vi "niFpga wdp fft tf 4096 U32 inv.vi"(4 "index":fxp<+,11,11>, 10 "enable":bool) -> (2 "imag":fxp<+/-,16,2>, 3 "real":fxp<+/-,16,2>)   [LabVIEW 2017]
uses:
  <vilib>/rvi/Emulation/niFpgaSctlEmulationGetInTimedLoop.vi
  <vilib>/Utility/error.llb/Clear Errors.vi
  <vilib>/rvi/DataTransferAndStorage/Container/Common/niFpgaContainerGetUniqueNameForEmu.vi
  <vilib>/rvi/DataTransferAndStorage/Container/Common/niFpgaContainerSetEmuInfo.vi
  <vilib>/rvi/eio/common/nirviEmuReportErrorAndStop.vi
  <vilib>/rvi/DataTransferAndStorage/Container/Common/niFpgaContainerExecOnDevCompGetState.vi
  <vilib>/rvi/Emulation/niFpgaEmulationIsFPGAContextNoSignature.vi
  <vilib>/rvi/Emulation/niFpgaProcessEmulError.vi
  <vilib>/rvi/errors/nirviReportUnexpectedCaseInternalError (U32).vi
  <vilib>/rvi/Memory/Memory_Emulation/niFpgaMemoryEmulationCacheClearOnFirstRun.vi
  <vilib>/rvi/Memory/Memory_Emulation/nirvimemoryEmulationManagerCache_MakeExclusive.vi
  <vilib>/rvi/Memory/Memory_Emulation/niFpgaMemoryEmulationValidateCache.vi
  <vilib>/rvi/Memory/Memory_Emulation/nirvimemoryEmulationManagerCache_InsertValue.vi
  <vilib>/rvi/Memory/Memory_Emulation/nirvimemoryEmulationManagerCache_ReleaseExclusive.vi
  <vilib>/rvi/Memory/Memory_Emulation/nirvimemoryEmulationManagerCache_GetValue.vi
  <vilib>/rvi/Memory/Memory_Emulation/nirvimemoryEmulationManagerCache_SetValue.vi
  <vilib>/rvi/Emulation/niFpgaSctlEmulationResourceMgr.vi
  <vilib>/rvi/LocalResourceManager/LocalResourceManager.xnode
  <vilib>/rvi/DataTransferAndStorage/Container/XNode/niFpgaContainer.xnode
  <vilib>/rvi/Memory/Memory_Emulation/niFpgaMemoryEmulationRefIn.vi
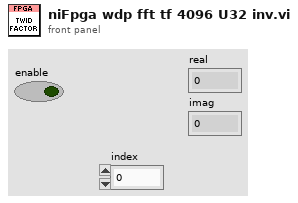
[diagram p1: front panel]
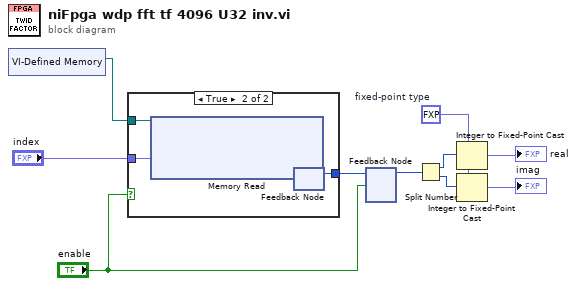
[diagram p0: block diagram]
diagram:
  w6 = fxp<+/-,16,2> 0.0  # fixed-point type
  n1 = xnode "VI-Defined Memory"() -> ("Memory Out"=w3:refnum<k21>)
  n2 = case shown="True" "enable" {
    tunnel: "index" -> [_ w13]
    tunnel: [_ w12] -> w9
    tunnel: w3 -> [_ w11]
    frame False {
    }
    frame True {
      n3 = xnode ("Memory Read")("Address"=w13, "Memory In"=w11) -> ("Data"=w14:u32)  [unwired: 1 out]
      n4 = feedback #1() -> (w12:u32)  [unwired: 1 in]
      n5 = feedback-in #1(w14) -> ()
    }
  }
  n6 = feedback #2() -> (w5:u32)  [unwired: 1 in]
  n7 = feedback-in #2(w9, "enable") -> ()
  n8 = Split Number(x=w5) -> (hi(x)=w8:u16, lo(x)=w7:u16)
  n9 = Integer to Fixed-Point Cast(fixed-point type=w6, integer=w8) -> (fixed-point=→"real":fxp<+/-,16,2>)
  n10 = Integer to Fixed-Point Cast(fixed-point type=w6, integer=w7) -> (fixed-point=→"imag":fxp<+/-,16,2>)
